vi "GT Get Control Superimposed.vi"(7 "pSuperimposedIndex":i16, 8 "error in (no error)":errorcluster caption="错误输入（无错误）", 9 "pSuperimposedType":i16, 10 "control":i16, 11 "cardNum":i16) -> (0 "error out":errorcluster caption="错误输出", 1 "pSuperimposedType out":i16, 3 "function return":i16, 5 "pSuperimposedIndex out":i16)   [LabVIEW 2014, in "gts.lvlib"]
doc: "GT_API GT_GetControlSuperimposed(short cardNum,short control,short *pSuperimposedType,short *pSuperimposedIndex);"
uses:
  gts.lvlib
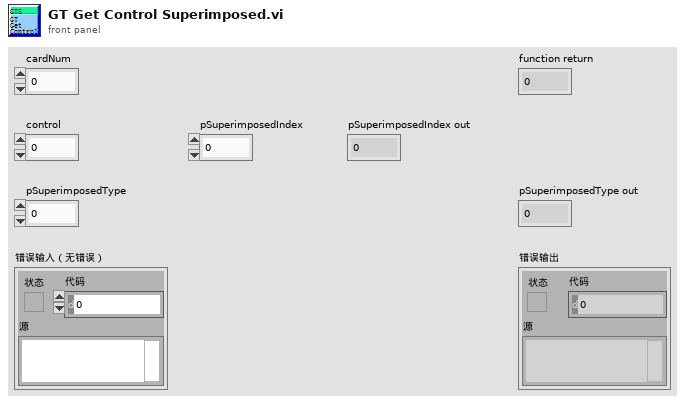
[diagram p1: front panel]
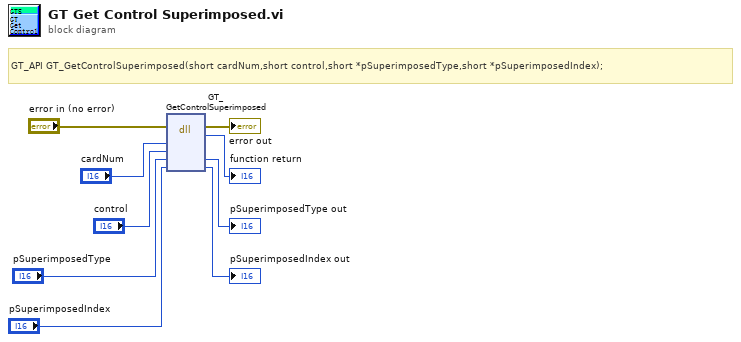
[diagram p0: block diagram]
diagram:
  # "GT_API GT_GetControlSuperimposed(short cardNum,short control,short *pSuperimposedType,short *pSuperimposedIndex);"
  n1 = dll-call lib="PTH2habs D固高科技资料GTS控制卡GTS卡18年上半年资料dllVC32bit\nmulti_cardgts.*" fn="GT_GetControlSuperimposed"(error in="error in (no error)", "cardNum"="cardNum", "control"="control", "pSuperimposedType"="pSuperimposedType", "pSuperimposedIndex"="pSuperimposedIndex") -> (error out=→"error out":errorcluster, →"function return":i16, "pSuperimposedType"=→"pSuperimposedType out":i16, "pSuperimposedIndex"=→"pSuperimposedIndex out":i16)  [unwired: 4 in, 1 out]
